vi "AWG Start Pulses.vi"(8 "error in (no error)":errorcluster, 11 "awg session in":T1={"type"=enum."Agilent 331xxA to 332xxA", "VISA"="", "enable 10MHz ref"=FALSE, "cmi ckd2"={"VISA"="", "clock source"=enum."Auto", "manual ref clk"=FALSE, "ref clock [Hz]"=0.0}, "cmi sync v3"={"VISA"="", "baud rate [bd/s]"=115200, "source"=enum."Auto", "hv range"=enum."1kV", "fsrc is fixed"=FALSE, "fsrc [Hz]"=10000000.0, "freq integ [s]"=1.0, "freq filter"=5, "trig level"=enum."TTL 5V", "chn1 mode"=enum."Source divider", "chn1 level"=enum."Positive 5V", "chn2 mode"=enum."Source divider", "chn2 level"=enum."Positive 5V", "chn2 div"=1, "chn3 mode"=enum."Chn 1 Active", "chn3 level"=enum."Positive 5V"}, "trigger"={"source"=enum."Immediate", "level [V]"=0.0, "coupling"=enum."DC", "slope"=enum."POS"}} {"cmi sync v3"."chn2 div" min=1 max=100000000 step=1; "cmi sync v3"."fsrc [Hz]" format="%_8p"}) -> (0 "error out":errorcluster, 3 "awg session out":T1={"type"=enum."Agilent 331xxA to 332xxA", "VISA"="", "enable 10MHz ref"=FALSE, "cmi ckd2"={"VISA"="", "clock source"=enum."Auto", "manual ref clk"=FALSE, "ref clock [Hz]"=0.0}, "cmi sync v3"={"VISA"="", "baud rate [bd/s]"=115200, "source"=enum."Auto", "hv range"=enum."1kV", "fsrc is fixed"=FALSE, "fsrc [Hz]"=10000000.0, "freq integ [s]"=1.0, "freq filter"=5, "trig level"=enum."TTL 5V", "chn1 mode"=enum."Source divider", "chn1 level"=enum."Positive 5V", "chn2 mode"=enum."Source divider", "chn2 level"=enum."Positive 5V", "chn2 div"=1, "chn3 mode"=enum."Chn 1 Active", "chn3 level"=enum."Positive 5V"}, "trigger"={"source"=enum."Immediate", "level [V]"=0.0, "coupling"=enum."DC", "slope"=enum."POS"}} {"cmi sync v3"."chn2 div" min=1 max=100000000 step=1; "cmi sync v3"."fsrc [Hz]" format="%_8p"})   [LabVIEW 2020, in "AWG.lvlib"]
doc: "AWG wrapper: Starts infinite pulse train with last set period."
uses:
  AWG.lvlib
  AWG Session.ctl
  AWG Type.ctl
  CMI Clock Divider v2/CMI ckd2 Session.ctl
  CMI Clock Divider v2/CMI ckd2 Source Mode.ctl
  CMI Sync V3/CMI Sync V3 session.ctl
  CMI Sync V3/Configure/CMI Sync V3 Reference Clock Source.ctl
  CMI Sync V3/Configure/CMI Sync V3 HV input Range.ctl
  CMI Sync V3/Configure/CMI Sync V3 Trigger Input Level.ctl
  CMI Sync V3/Configure/CMI Sync V3 Channel 1 Mode.ctl
  CMI Sync V3/Configure/CMI Sync V3 Channel Output Levels.ctl
  CMI Sync V3/Configure/CMI Sync V3 Channel 2 Mode.ctl
  CMI Sync V3/Configure/CMI Sync V3 Channel 3 Mode.ctl
  CMI Sync V3/Configure/CMI Sync V3 Trigger Mode.ctl
  Agilent 33XXX Series/Agilent 33XXX Series.lvlib
  CMI Sync V3/CMI Sync Unit V3.lvlib
  adc/ADC Trig Slope.ctl
  adc/ADC Trig Mode Source.ctl
  adc/ADC Trig Coupling.ctl
  adc/ADC Trig Config.ctl
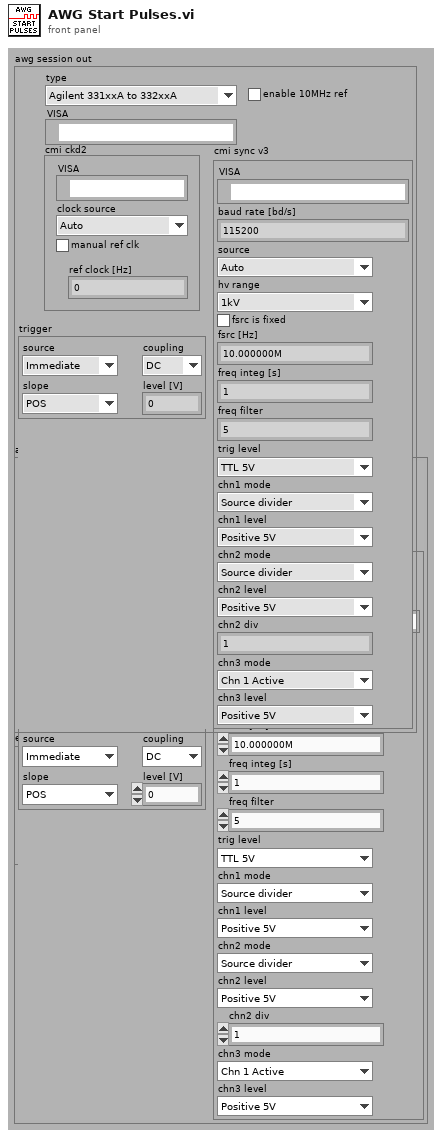
[diagram p1: front panel]
types:
  T1 = typedef "AWG.lvlib/AWG Session.ctl" = cluster{"type":T2, "VISA":refnum<visa-resource-name>, "enable 10MHz ref":bool, "cmi ckd2":T3, "cmi sync v3":T5, "trigger":T13}
  T2 = typedef "AWG.lvlib/AWG Type.ctl" = enum16{"Agilent 331xxA to 332xxA", "Agilent 335xxA to 336xxA", "Tektronix AFG3101C", "CMI Clock Divider v2", "CMI Sync Unit V3", "dummy"}
  T3 = typedef "AWG.lvlib/CMI ckd2 Session.ctl" = cluster{"VISA":refnum<visa-resource-name>, "clock source":T4, "manual ref clk":bool, "ref clock [Hz]":dbl}
  T4 = typedef "AWG.lvlib/CMI ckd2 Source Mode.ctl" = enum16{"Auto", "LF clock", "HF clock", "Internal"}
  T5 = typedef "AWG.lvlib/CMI Sync Unit V3.lvlib/CMI Sync V3 session.ctl" = cluster{"VISA":refnum<visa-resource-name>, "baud rate [bd/s]":i32, "source":T6, "hv range":T7, "fsrc is fixed":bool, "fsrc [Hz]":dbl, "freq integ [s]":dbl, "freq filter":i32, "trig level":T8, "chn1 mode":T9, "chn1 level":T10, "chn2 mode":T11, "chn2 level":T10, "chn2 div":i32, "chn3 mode":T12, "chn3 level":T10}
  T6 = typedef "AWG.lvlib/CMI Sync Unit V3.lvlib/CMI Sync V3 Reference Clock Source.ctl" = enum16{"Auto", "Internal", "Logic", "Sine", "HV"}
  T7 = typedef "AWG.lvlib/CMI Sync Unit V3.lvlib/CMI Sync V3 HV input Range.ctl" = enum16{"10V", "60V", "250V", "1kV"}
  T8 = typedef "AWG.lvlib/CMI Sync Unit V3.lvlib/CMI Sync V3 Trigger Input Level.ctl" = enum16{"LVCMOS 3V3", "TTL 5V"}
  T9 = typedef "AWG.lvlib/CMI Sync Unit V3.lvlib/CMI Sync V3 Channel 1 Mode.ctl" = enum16{"Source divider", "DDS absolute", "DDS ratio", "DDS ratio M/N"}
  T10 = typedef "AWG.lvlib/CMI Sync Unit V3.lvlib/CMI Sync V3 Channel Output Levels.ctl" = enum16{"Positive 3V3", "Negative 3V3", "Positive 5V", "Negative 5V"}
  T11 = typedef "AWG.lvlib/CMI Sync Unit V3.lvlib/CMI Sync V3 Channel 2 Mode.ctl" = enum16{"Source divider", "Chn 1 divide"}
  T12 = typedef "AWG.lvlib/CMI Sync Unit V3.lvlib/CMI Sync V3 Channel 3 Mode.ctl" = enum16{"Chn 1 Active", "Chn 2 Active", "Chn 1 Trigger", "Chn 2 Trigger", "Gate", "PPS", "10MHz"}
  T13 = typedef "ADC Trig Config.ctl" = cluster{"source":T14, "level [V]":dbl, "coupling":T15, "slope":T16}
  T14 = typedef "ADC Trig Mode Source.ctl" = enum16{"Immediate", "External", "Level"}
  T15 = typedef "ADC Trig Coupling.ctl" = enum16{"DC", "AC"}
  T16 = typedef "ADC Trig Slope.ctl" = enum16{"POS", "NEG"}
  T17 = typedef "AWG.lvlib/CMI Sync Unit V3.lvlib/CMI Sync V3 Trigger Mode.ctl" = enum16{"Hold", "Auto (continuous)", "Gate positive", "Gate negative", "Rising edge", "Falling edge", "Bus (*TRG)", "Manual (button)"}
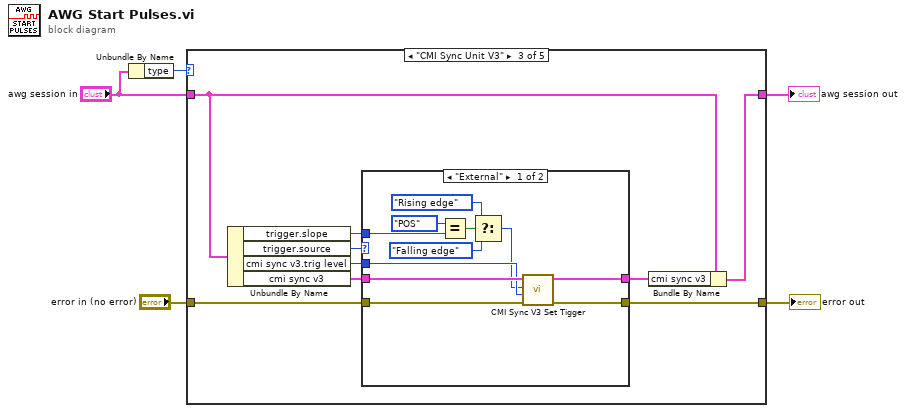
[diagram p0: block diagram]
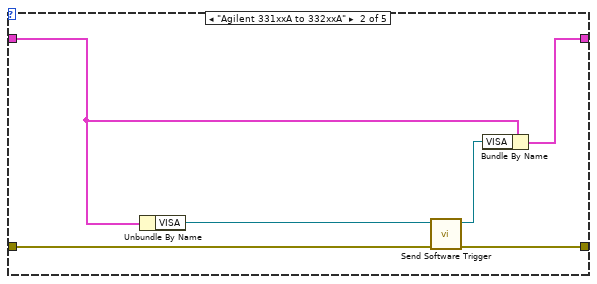
[diagram p3: hidden frame]
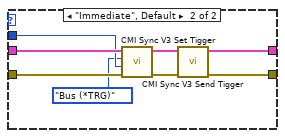
[diagram p4: hidden frame]
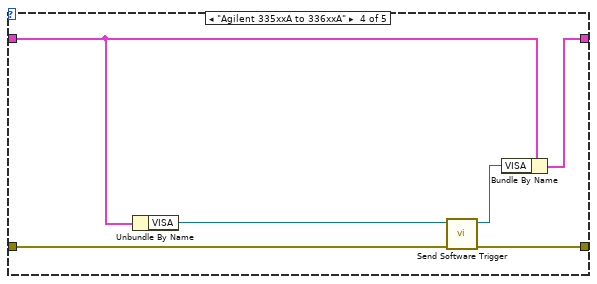
[diagram p5: hidden frame]
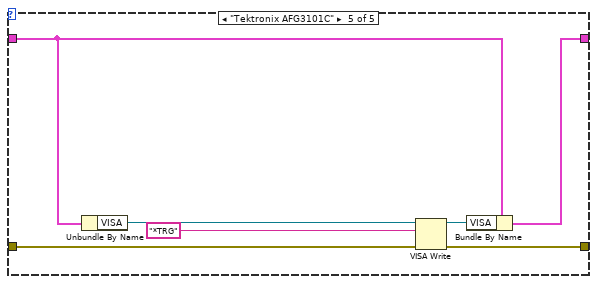
[diagram p6: hidden frame]
diagram:
  n1 = Unbundle By Name("awg session in") -> ("type"=w5:T2)
  n2 = case shown="\"CMI Sync Unit V3\"" w5 {
    tunnel: "error in (no error)" -> [w7 w8 w16 w42 w49]
    tunnel: [w7 w11 w19 w44 w54] -> w3
    tunnel: "awg session in" -> [w6 w12 w22 w47 w53]
    tunnel: [w6 w13 w21 w46 w50] -> w1
    frame Default {
    }
    frame "Agilent 331xxA to 332xxA" {
      n3 = Unbundle By Name(w12) -> ("VISA"=w9:refnum<visa-resource-name>)
      n4 = call "Send Software Trigger.vi"("error in (no error)"=w8, "VISA resource name"=w9) -> ("error out"=w11:errorcluster, "VISA resource name out"=w10:refnum<visa-resource-name>)  [unwired: 8 in]
      n5 = Bundle By Name(cluster=w12, "VISA"=w10) -> (w13:T1)
    }
    frame "CMI Sync Unit V3" {
      n6 = Unbundle By Name(w22) -> ("trigger.slope"=w14:T16, "trigger.source"=w15:T14, "cmi sync v3.trig level"=w17:T8, "cmi sync v3"=w18:T5)
      n7 = case shown="\"External\"" w15 {
        tunnel: [w23 w41] -> w20
        tunnel: [w24 w40] -> w19
        tunnel: w18 -> [w33 w37]
        tunnel: w17 -> [w32 w36]
        tunnel: w16 -> [w31 w35]
        tunnel: w14 -> [w30 _]
        frame "External" {
          n8 = Equal?(x=ADC_Trig_Slope."POS", y=w30) -> (x = y?=w28:bool)
          n9 = Select(t=CMI_Sync_V3_Trigger_Mode."Rising edge" ("Trigger mode (Auto)"), s=w28, f=CMI_Sync_V3_Trigger_Mode."Falling edge" ("Trigger mode (Auto)")) -> (s? t:f=w27:T17)
          n10 = call "CMI Sync V3 Set Tigger.vi"("error in"=w31, "Trigger input logic (5V)"=w32, "Trigger mode (Auto)"=w27, "session in"=w33) -> ("error out"=w24:errorcluster, "session out"=w23:T5)  [unwired: 6 in]
        }
        frame "Immediate", Default {
          n11 = call "CMI Sync V3 Set Tigger.vi"("error in"=w35, "Trigger input logic (5V)"=w36, "Trigger mode (Auto)"=CMI_Sync_V3_Trigger_Mode."Bus (*TRG)", "session in"=w37) -> ("error out"=w39:errorcluster, "session out"=w38:T5)  [unwired: 6 in]
          n12 = call "CMI Sync V3 Send Tigger.vi"("error in"=w39, "session in"=w38) -> ("error out"=w40:errorcluster, "session out"=w41:T5)  [unwired: 8 in]
        }
      }
      n13 = Bundle By Name(cluster=w22, "cmi sync v3"=w20) -> (w21:T1)
    }
    frame "Agilent 335xxA to 336xxA" {
      n14 = Unbundle By Name(w47) -> ("VISA"=w43:refnum<visa-resource-name>)
      n15 = call "Send Software Trigger.vi"("error in (no error)"=w42, "VISA resource name"=w43) -> ("error out"=w44:errorcluster, "VISA resource name out"=w45:refnum<visa-resource-name>)  [unwired: 8 in]
      n16 = Bundle By Name(cluster=w47, "VISA"=w45) -> (w46:T1)
    }
    frame "Tektronix AFG3101C" {
      n17 = Unbundle By Name(w53) -> ("VISA"=w48:refnum<visa-resource-name>)
      n18 = VISA Write(VISA resource name=w48, write buffer="*TRG", error in (no error)=w49) -> (VISA resource name out=w52:refnum<visa-resource-name>, error out=w54:errorcluster)  [unwired: 1 out]
      n19 = Bundle By Name(cluster=w53, "VISA"=w52) -> (w50:T1)
    }
  }
  "error out" <- w3
  "awg session out" <- w1
